vi "check_and_correct_input.vi"(4 "delay array":dbl[](array[numeric])) -> (1 "corrrected delay array":dbl[](array[numeric]))   [LabVIEW 2012]
doc: "Check if all the values entered by the user are correct. See the block diagram for the rules and add some if need be. \nThis vi also makes noise and shows the user what he did wrong!"
panel:
  # "check for correct data entry, \ncorrect data if necessary,\n play sound if input was wrong \nand show what was wrong"
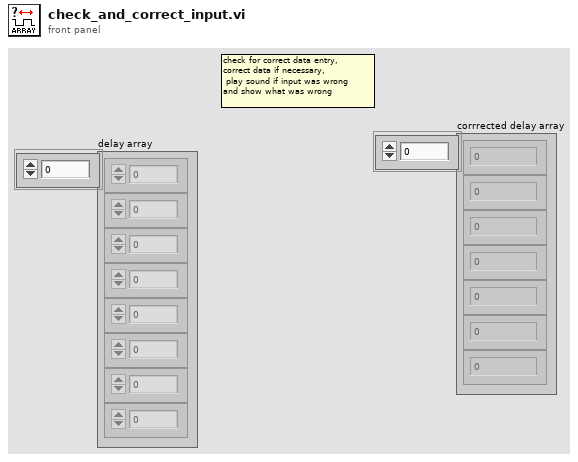
[diagram p1: front panel]
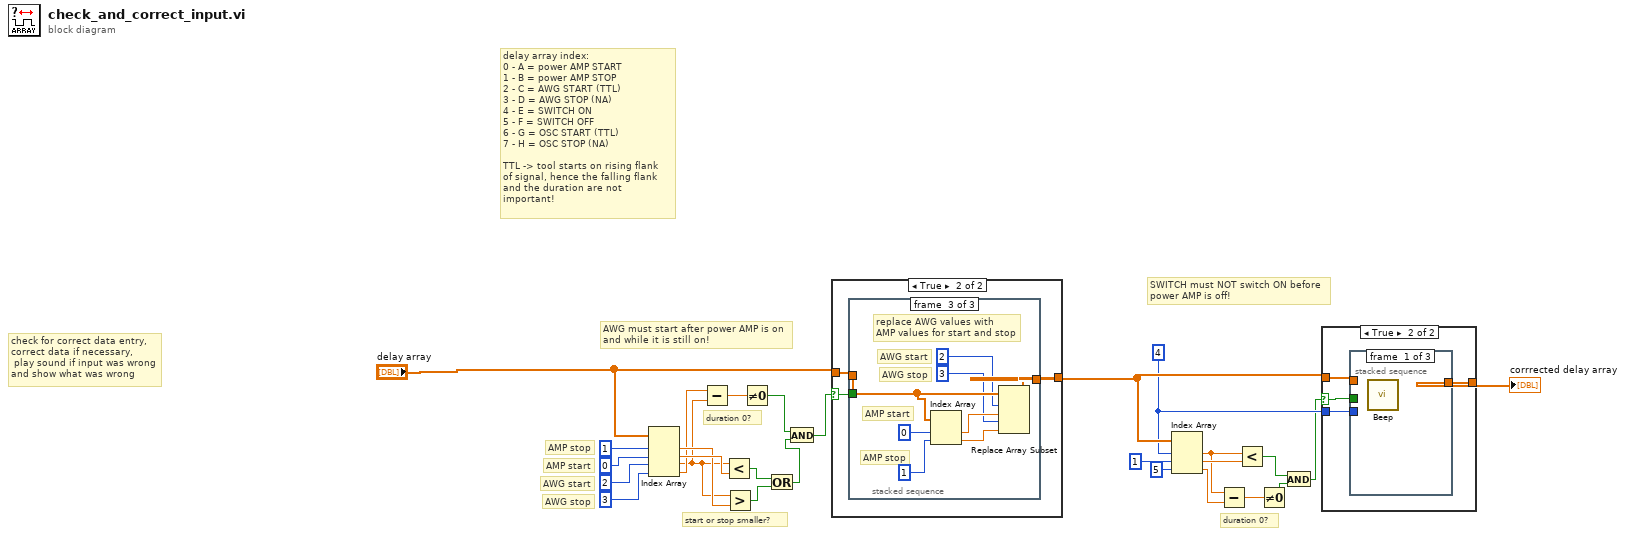
[diagram p0: block diagram]
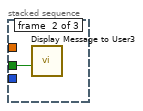
[diagram p3: hidden frame]
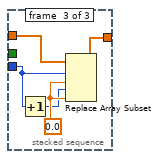
[diagram p4: hidden frame]
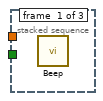
[diagram p6: hidden frame]
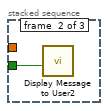
[diagram p7: hidden frame]
diagram:
  w10 = 4 ("index")
  # "duration 0?"
  # "SWITCH must NOT switch ON before \npower AMP is off!"
  # "start or stop smaller?"
  # "AWG stop"
  # "AWG start"
  # "AMP stop"
  # "AMP start"
  # "duration 0?"
  # "AWG must start after power AMP is on \nand while it is still on!"
  # "check for correct data entry, \ncorrect data if necessary,\n play sound if input was wrong \nand show what was wrong"
  # "delay array index:\n0 - A = power AMP START\n1 - B = power AMP STOP\n2 - C = AWG START (TTL)\n3 - D = AWG STOP (NA)\n4 - E = SWITCH ON \n5 - F = SWITCH OFF\n6 - G = OSC START (TTL)\n7 - H = OSC STOP (NA)\n\nTTL -> tool starts on rising flank\nof signal, hence the falling flank \nand the duration are not important!"
  n1 = Index Array(array="delay array", index #1=1 ("index"), index #2=0 ("index"), index #3=2 ("index"), index #4=3 ("index")) -> (element #1=w19:dbl, element #2=w20:dbl, element #3=w12:dbl, element #4=w13:dbl)
  n2 = Subtract(x=w13, y=w12) -> (x-y=w23:dbl)
  n3 = Less?(x=w12, y=w20) -> (x < y?=w18:bool)
  n4 = Greater?(x=w12, y=w19) -> (0:w17:bool)
  n5 = Not Equal To 0?(x=w23) -> (x != 0?=w16:bool)
  n6 = Or(x=w18, y=w17) -> (x .or. y?=w15:bool)
  n7 = And(x=w16, y=w15) -> (x .and. y?=w14:bool)
  n8 = case shown="True" w14 {
    selector: w14 -> [_ w31]
    tunnel: [w28 w30] -> w27
    tunnel: "delay array" -> [w28 w29]
    frame False {
    }
    frame True {
      n9 = stacked-sequence {
        tunnel: w31 -> [_ w32 _]
        tunnel: [_ _ w40] -> w30
        tunnel: w29 -> [_ _ w37]
        frame #0 {
          n10 = call <vilib>:"Beep.vi"() -> ()  [unwired: 12 in]
        }
        frame #1 {
          n11 = call "Display Message to User2"("Enable"=w32) -> ()  [unwired: 9 in, 2 out]
        }
        frame #2 {
          # "replace AWG values with \nAMP values for start and stop"
          # "AWG stop"
          # "AWG start"
          # "AMP start"
          # "AMP stop"
          n12 = Index Array(array=w37, index #1=0 ("index"), index #2=1 ("index")) -> (element #1=w35:dbl, element #2=w34:dbl)
          n13 = Replace Array Subset(array=w37, new element #1=w35, index #1=2 ("index"), new element #2=w34, index #2=3 ("index")) -> (w40:dbl[])
        }
      }
    }
  }
  n14 = Index Array(array=w27, index #1=w10, index #2=1 ("index"), index #3=5 ("index")) -> (element #1=w7:dbl, element #2=w9:dbl, element #3=w6:dbl)
  n15 = Subtract(x=w7, y=w6) -> (x-y=w5:dbl)
  n16 = Less?(x=w7, y=w9) -> (x < y?=w3:bool)
  n17 = Not Equal To 0?(x=w5) -> (x != 0?=w4:bool)
  n18 = And(x=w3, y=w4) -> (x .and. y?=w2:bool)
  n19 = case shown="True" w2 {
    selector: w2 -> [_ w45]
    tunnel: [w41 w44] -> w26
    tunnel: w27 -> [w41 w43]
    tunnel: w10 -> [_ w42]
    frame False {
    }
    frame True {
      n20 = stacked-sequence {
        tunnel: w45 -> [_ w46 _]
        tunnel: [_ _ w51] -> w44
        tunnel: w43 -> [_ _ w49]
        tunnel: w42 -> [_ _ w48]
        frame #0 {
          n21 = call <vilib>:"Beep.vi"() -> ()  [unwired: 12 in]
        }
        frame #1 {
          n22 = call "Display Message to User3"("Enable"=w46) -> ()  [unwired: 9 in, 2 out]
        }
        frame #2 {
          w50 = 0.0 ("new element/subarray")
          n23 = Increment(x=w48) -> (x+1=w47:i32)
          n24 = Replace Array Subset(array=w49, new element #1=w50, index #1=w48, new element #2=w50, index #2=w47) -> (w51:dbl[])
        }
      }
    }
  }
  "corrrected delay array" <- w26
